vi "main.vi"() -> ()   [LabVIEW 2017]
uses:
  <vilib>/MakerHub/LINX/Public/Utilities/Open Serial.vi
  <vilib>/MakerHub/LINX/LMH-LINX.lvlib
panel:
  out "串口指示灯":bool
  out "成绩表":string[][](table)
  out "布尔":bool
  in  "硬件端口":refnum<visa-resource-name>="COM4"
  out "led1":bool
  out "黄绿色":bool
  out "绿色":bool
  out "蓝绿色":bool
  out "蓝色":bool
  out "蓝紫色":bool
  out "紫色":bool
  out "红紫色":bool
  out "品红":bool
  out "橙红色":bool
  out "橙色":bool
  out "黄橙色":bool
  out "黄色":bool
  out "led 12":bool
  out "led 11":bool
  out "led 10":bool
  out "led 9":bool
  out "led 8":bool
  out "led 7":bool
  out "led 6":bool
  out "led 5":bool
  out "led 4":bool
  out "led 3":bool
  out "led 2":bool
  out "Error Out":errorcluster
  out "B coff":dbl format="%.6f"
  out "G coff":dbl format="%.6f"
  out "R coff":dbl format="%.6f"
  in  "CAL":bool
  in  "学号":string="17101130123"
  in  "班级":string="视觉172"
  out "姓名":string
  in  "全体结束":bool
  in  "个人结束":bool
  in  "初始化":bool
  out "Blue":u8
  out "Green":u8
  out "Red":u8
  out "已答题数":u8(slide) scale=0.0..12.0
  out "stdcolour":u32[](array[colorbox])
  in  "boolcolour":bool[](array[boolean])
  out "error out":errorcluster caption="错误输出"
  in  "error in (no error)":errorcluster caption="错误输入（无错误）"
  out "已得分数":u8(slide) scale=0.0..100.0
  out "Color":u32(colorbox) caption="颜色"
  # "基于LabVIEW与颜色传感器的色环检测系统"
  # "黄色"
  # "黄橙色"
  # "橙色"
  # "橙红色"
  # "品红"
  # "红紫色"
  # "紫色"
  # "蓝紫色"
  # "蓝色"
  # "蓝绿色"
  # "绿色"
  # "黄绿色"
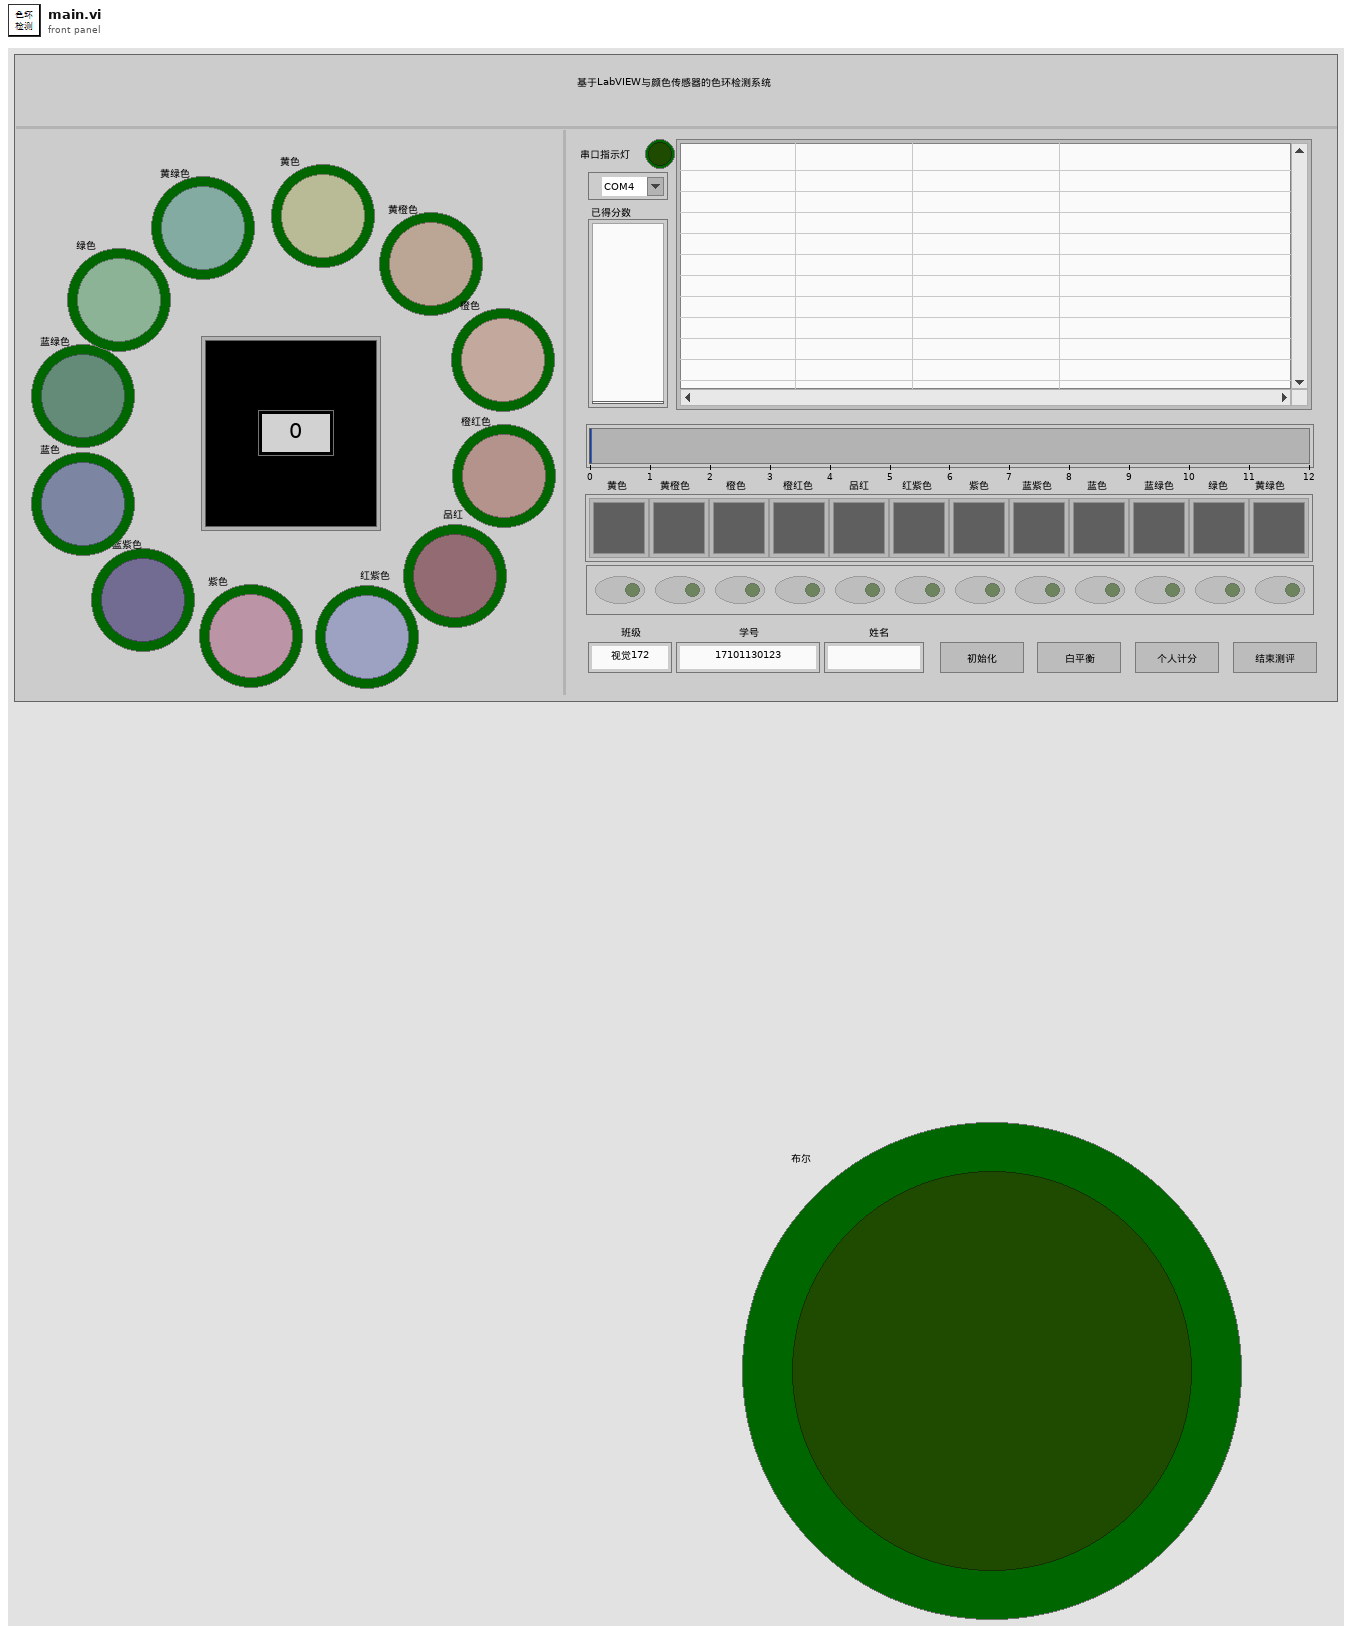
[diagram p1: front panel]
types:
  T1 = enum16{"open", "replace", "create", "open or create", "replace or create", "replace or create with confirmation"}
  T2 = typedef "LMH-LINX.lvlib/LINX Ref.ctl" = cluster{"IO":T3, "Interface":T4, "LINX Device Config":T5}
  T3 = typedef "LMH-LINX.lvlib/Platform.ctl" = enum16{"Remote", "Local"}
  T4 = typedef "LMH-LINX.lvlib/Interface.ctl" = enum16{"Serial", "TCP"}
  T5 = typedef "LMH-LINX.lvlib/Device.lvlib/LINX Device Config.ctl" = cluster{"Interface":T4, "COM Port":refnum<visa-resource-name>, "TCP Configuration":T6, "Device Family":u8, "Device ID":u8, "Device Name":string, "TCP Ref":refnum<k5>, "Channels":T7}
  T6 = typedef "LMH-LINX.lvlib/Device.lvlib/TCP Config.ctl" = cluster{"IP Address":string, "Port":u16}
  T7 = typedef "LMH-LINX.lvlib/Channels.ctl" = cluster{"DI":u8[], "DO":u8[], "AI":u8[], "AO":u8[], "PWM":u8[], "QE":u8[], "UART":u8[], "I2C 2":u8[], "SPI":u8[], "CAN":u8[], "Servo":u8[], "AI Ref (V)":dbl, "AI Resolution (Bits)":u8, "AO Ref (V)":dbl, "AO Resolution (Bits)":u8}
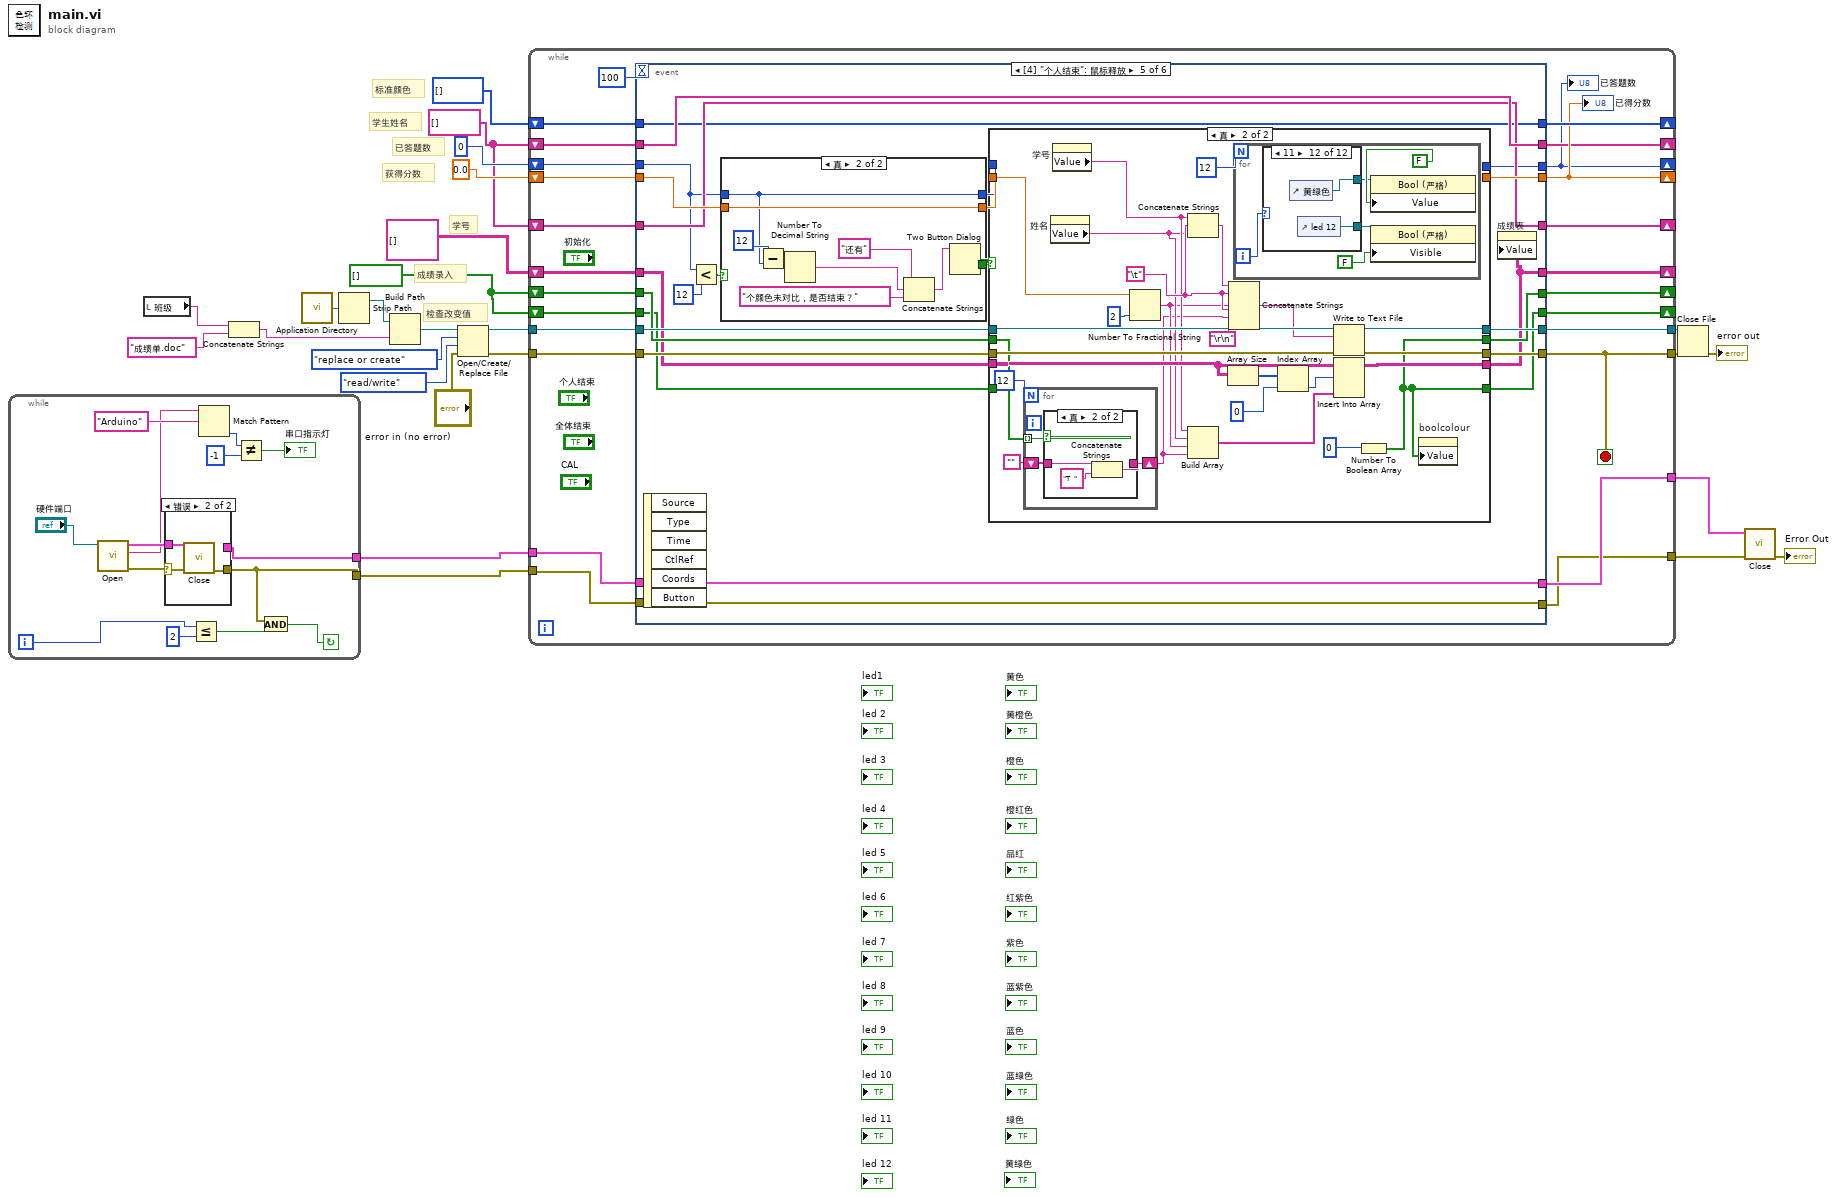
[diagram p0: block diagram]
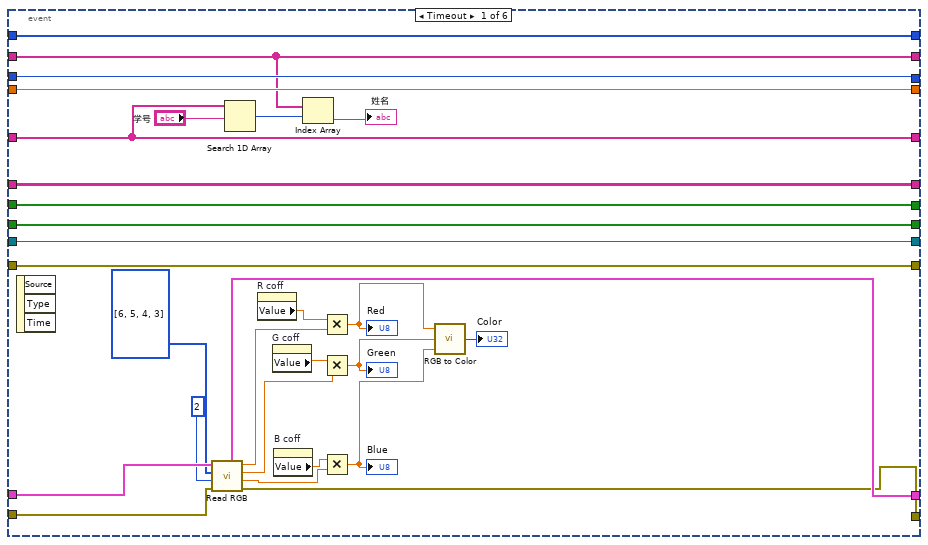
[diagram p3: hidden frame]
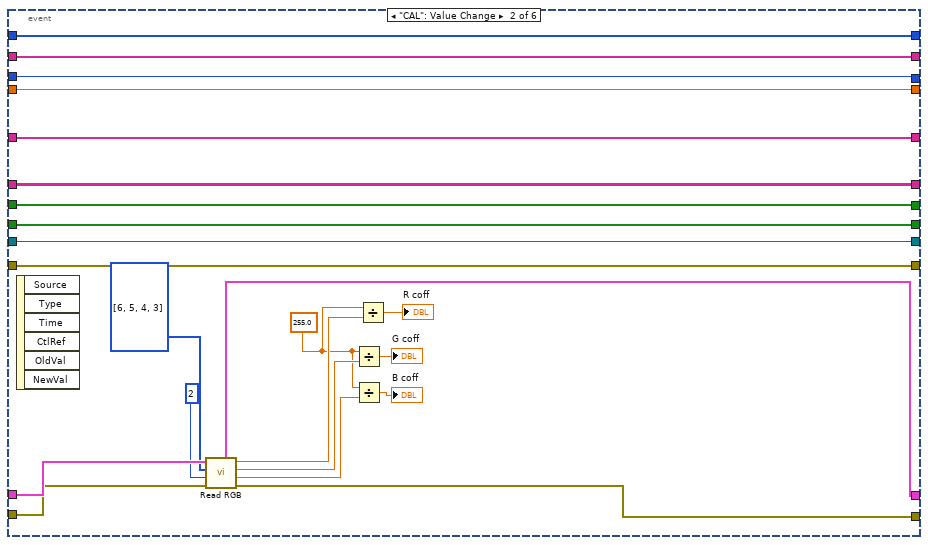
[diagram p4: hidden frame]
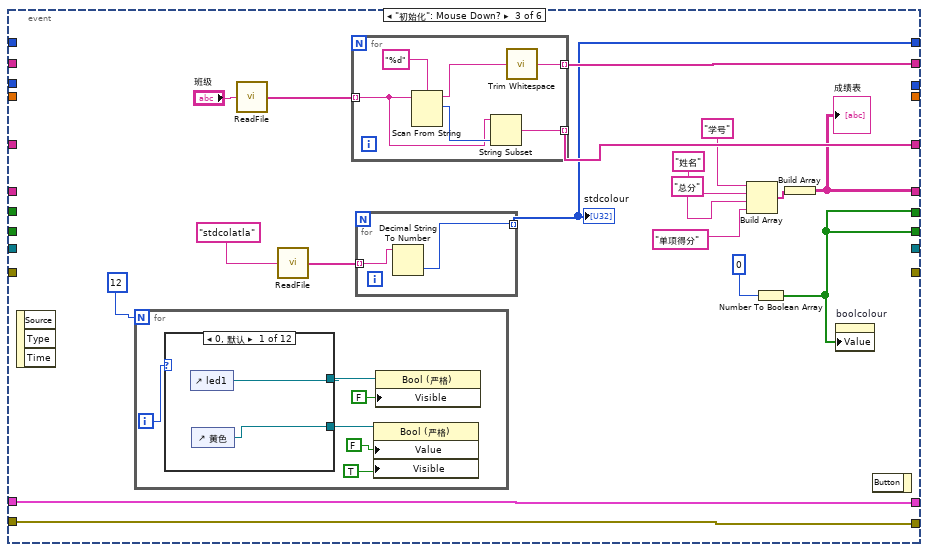
[diagram p5: hidden frame]
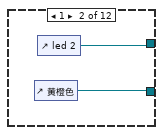
[diagram p6: hidden frame]
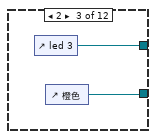
[diagram p7: hidden frame]
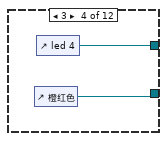
[diagram p8: hidden frame]
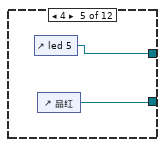
[diagram p9: hidden frame]
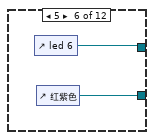
[diagram p10: hidden frame]
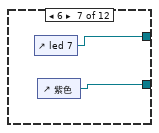
[diagram p11: hidden frame]
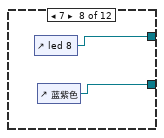
[diagram p12: hidden frame]
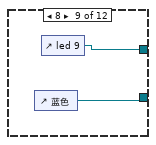
[diagram p13: hidden frame]
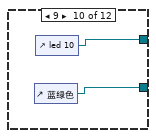
[diagram p14: hidden frame]
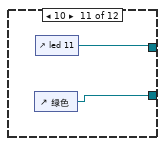
[diagram p15: hidden frame]
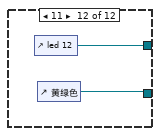
[diagram p16: hidden frame]
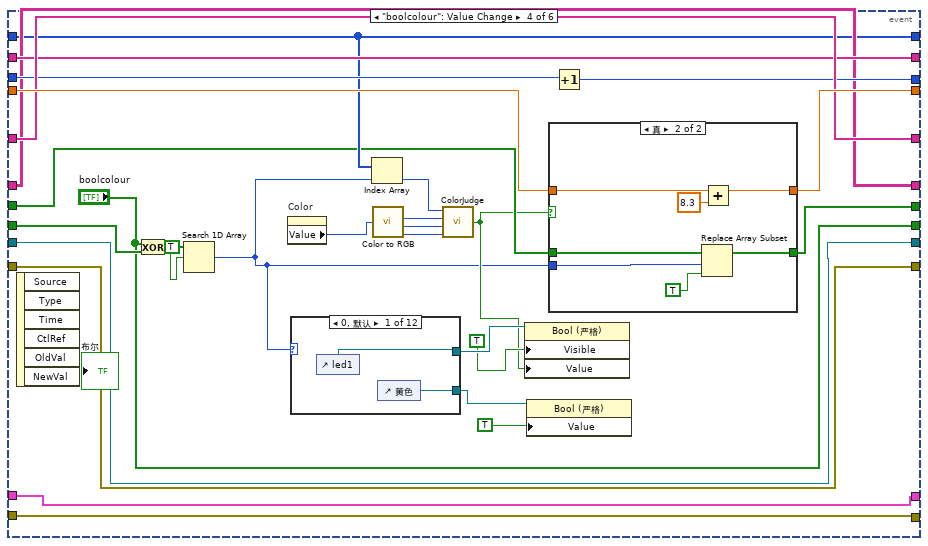
[diagram p17: hidden frame]
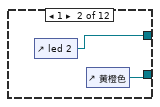
[diagram p18: hidden frame]
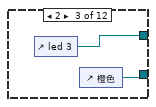
[diagram p19: hidden frame]
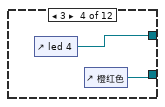
[diagram p20: hidden frame]
diagram:
  w10 = bool[] []
  w11 = string[] []
  # "检查改变值"
  # "成绩录入"
  # "已答题数"
  # "学号"
  # "获得分数"
  # "学生姓名"
  # "标准颜色"
  n1 = while {
    tunnel: [w36] -> w8
    tunnel: [w35] -> w5
    i -> [w34]
    stop <- w31 continue-if-true
    n2 = call-poly <vilib>:"Open.vi"("Serial Port"="硬件端口") -> ("Error Out"=w38:errorcluster, "Device Name"=w27:string, "LINX Resource"=w37:T2)  [unwired: 8 in]
    n3 = case shown="错误" w38 {
      selector: w38 -> [w40 w43]
      tunnel: w37 -> [w41 w42]
      tunnel: [w41 _] -> w36
      tunnel: [w40 w44] -> w35
      frame No Error {
      }
      frame Error {
        n4 = call <vilib>:"Close.vi"("Error In"=w43, "LINX Resource"=w42) -> ("Error Out"=w44:errorcluster)  [unwired: 9 in]
      }
    }
    n5 = Less Or Equal?(x=w34, y=2) -> (x <= y?=w32:bool)
    n6 = Match Pattern(string=w27, regular expression="Arduino" ("格式字符串")) -> (offset past match=w29:i32)  [unwired: 1 in, 3 out]
    n7 = Not Equal?(x=w29, y=-1) -> (x != y?=→"串口指示灯":bool)
    n8 = And(x=w35, y=w32) -> (x .and. y?=w31:bool)
  }
  n9 = local read "班级"() -> (w3:string)
  n10 = Concatenate Strings(w3, "成绩单.doc" ("名称或相对路径")) -> (w1:string)
  n11 = call <vilib>:"Application Directory.vi"() -> ("Application Directory"=w24:path)
  n12 = Strip Path(path=w24) -> (stripped path=w23:path)  [unwired: 1 out]
  n13 = Build Path(base path=w23, name or relative path=w1) -> (appended path=w22:path)
  n14 = Open/Create/Replace File(file path (use dialog)=w22, error in="error in (no error)", operation (0:open)=T1."replace or create" ("操作(0:open)"), access (0:read/write)=enum16{"read/write", "read-only", "write-only"}."read/write" ("权限(0:read/write)")) -> (refnum out=w19:refnum<file>, error out=w18:errorcluster)  [unwired: 2 in, 1 out]
  n15 = while {
    shift-right: [w69] -> _
    shift-left: i32[] [] -> [w68]
    tunnel: w19 -> [w51]
    tunnel: w18 -> [w67]
    tunnel: [w65] -> w16
    tunnel: [w66] -> w17
    shift-right: [w63] -> _
    shift-left: 0.0 -> [w64]
    shift-right: [w61] -> _
    shift-left: w11 -> [w60]
    shift-right: [w62] -> _
    shift-left: w11 -> [w59]
    shift-right: [w57] -> _
    shift-left: w10 -> [w58]
    shift-right: [w52] -> _
    shift-left: 0 -> [w56]
    shift-right: [w45] -> _
    shift-left: string[][] [] -> [w55]
    shift-right: [w53] -> _
    shift-left: w10 -> [w54]
    tunnel: w8 -> [w50]
    tunnel: [w49] -> w7
    tunnel: [w48] -> w6
    tunnel: w5 -> [w47]
    stop <- w66 stop-if-true
    n16 = event shown="[4] \"个人结束\": 鼠标释放" {
      selector: _ -> [_ _ _ _ _ _]
      dyn-events: _ -> [_ _ _ _ _ _]
      timeout: 100 -> [_ _ _ _ _ _]
      tunnel: [w98 w121 w133 w191 w243 _] -> w69
      tunnel: w68 -> [w98 w121 _ w191 w243 _]
      tunnel: w67 -> [w91 w112 _ w192 w262 _]
      tunnel: [w91 w112 _ w192 w261 errorcluster {"status"=TRUE, "code"=0, "source"=""} ("error in (no error) 2")] -> w66
      tunnel: [w92 w113 _ w193 w260 _] -> w65
      tunnel: w51 -> [w92 w113 _ w193 w259 _]
      tunnel: w64 -> [w96 w118 _ w203 w255 _]
      tunnel: [w96 w118 _ w202 w257 _] -> w63
      tunnel: [w71 w120 w137 w200 w253 _] -> w61
      tunnel: [w73 w117 w136 w201 w252 _] -> w62
      tunnel: w60 -> [w71 w120 _ w200 w253 _]
      tunnel: w59 -> [w73 w117 _ w201 w252 _]
      tunnel: w58 -> [w94 w115 _ w189 w251 _]
      tunnel: [w94 w115 w125 w188 w250 _] -> w57
      tunnel: w56 -> [w97 w119 _ w199 w249 _]
      tunnel: [w97 w119 _ w198 w248 _] -> w52
      tunnel: w55 -> [w95 w116 _ w197 w246 w349]
      tunnel: [w95 w116 w122 w197 w240 w349] -> w45
      tunnel: w54 -> [w93 w114 _ w196 w245 _]
      tunnel: [w93 w114 w125 "boolcolour" w244 _] -> w53
      tunnel: w50 -> [w83 w104 w124 w183 w242 w348]
      tunnel: [w80 w100 w124 w183 w242 w348] -> w49
      tunnel: [w79 w99 w123 w182 w241 w347] -> w48
      tunnel: w47 -> [w78 w103 w123 w182 w241 w347]
      event Timeout {
        n17 = event-data() -> ()  [unwired: 1 in, 3 out]
        n18 = call "Read RGB.vi"("错误输入（无错误）"=w78, "Pulse OUT"=u8 2, "S0S1S2S3"=u8[] [6, 5, 4, 3] ("DO Channels"), "LINX Resource输入"=w83) -> ("错误输出"=w79:errorcluster, "Blue"=w88:dbl, "Green"=w89:dbl, "Red"=w90:dbl, "LINX Resource输出"=w80:T2)  [unwired: 3 in]
        n19 = Search 1D Array(1D array=w73, element="学号") -> (index of element=w72:i32)  [unwired: 1 in]
        n20 = property on="R coff" class="DigNum (严格)"() -> ("Value"=w77:dbl)  [unwired: 2 in, 2 out]
        n21 = property on="G coff" class="DigNum (严格)"() -> ("Value"=w76:dbl)  [unwired: 2 in, 2 out]
        n22 = property on="B coff" class="DigNum (严格)"() -> ("Value"=w75:dbl)  [unwired: 2 in, 2 out]
        n23 = Index Array(array=w71, index=w72) -> (element=→"姓名":string)
        n24 = Multiply(x=w77, y=w90) -> (x*y=w86:dbl)
        "Red" <- w86
        n25 = Multiply(x=w76, y=w89) -> (x*y=w85:dbl)
        "Green" <- w85
        n26 = Multiply(x=w75, y=w88) -> (x*y=w84:dbl)
        "Blue" <- w84
        n27 = call <vilib>:"RGB to Color.vi"("B"=w84, "G"=w85, "R"=w86) -> ("Color"=→"Color":u32)
      }
      event "CAL": Value Change {
        w108 = 255.0 ("x")
        n28 = event-data() -> ()  [unwired: 1 in, 6 out]
        n29 = call "Read RGB.vi"("错误输入（无错误）"=w103, "Pulse OUT"=u8 2, "S0S1S2S3"=u8[] [6, 5, 4, 3] ("DO Channels"), "LINX Resource输入"=w104) -> ("错误输出"=w99:errorcluster, "Blue"=w109:dbl, "Green"=w110:dbl, "Red"=w111:dbl, "LINX Resource输出"=w100:T2)  [unwired: 3 in]
        n30 = Divide(x=w108, y=w110) -> (x/y=→"G coff":dbl)
        n31 = Divide(x=w108, y=w109) -> (x/y=→"B coff":dbl)
        n32 = Divide(x=w108, y=w111) -> (x/y=→"R coff":dbl)
      }
      event "初始化": Mouse Down? {
        n33 = event-data() -> ()  [unwired: 1 in, 3 out]
        n34 = for {
          N: 12 -> [_]
          i -> [w145]
          n35 = case shown="0, 默认" w145 {
            tunnel: [w147 w149 w151 w153 w155 w157 w159 w161 w163 w165 w167 w169] -> w144
            tunnel: [w146 w148 w150 w152 w154 w156 w158 w160 w162 w164 w166 w168] -> w142
            frame 0, Default {
              n36 = control-ref of="led1"() -> (w147:refnum<vi>)
              n37 = control-ref of="黄色"() -> (w146:refnum<vi>)
            }
            frame 1 {
              n38 = control-ref of="黄橙色"() -> (w148:refnum<vi>)
              n39 = control-ref of="led 2"() -> (w149:refnum<vi>)
            }
            frame 2 {
              n40 = control-ref of="led 3"() -> (w151:refnum<vi>)
              n41 = control-ref of="橙色"() -> (w150:refnum<vi>)
            }
            frame 3 {
              n42 = control-ref of="橙红色"() -> (w152:refnum<vi>)
              n43 = control-ref of="led 4"() -> (w153:refnum<vi>)
            }
            frame 4 {
              n44 = control-ref of="led 5"() -> (w155:refnum<vi>)
              n45 = control-ref of="品红"() -> (w154:refnum<vi>)
            }
            frame 5 {
              n46 = control-ref of="led 6"() -> (w157:refnum<vi>)
              n47 = control-ref of="红紫色"() -> (w156:refnum<vi>)
            }
            frame 6 {
              n48 = control-ref of="led 7"() -> (w159:refnum<vi>)
              n49 = control-ref of="紫色"() -> (w158:refnum<vi>)
            }
            frame 7 {
              n50 = control-ref of="led 8"() -> (w161:refnum<vi>)
              n51 = control-ref of="蓝紫色"() -> (w160:refnum<vi>)
            }
            frame 8 {
              n52 = control-ref of="蓝色"() -> (w162:refnum<vi>)
              n53 = control-ref of="led 9"() -> (w163:refnum<vi>)
            }
            frame 9 {
              n54 = control-ref of="蓝绿色"() -> (w164:refnum<vi>)
              n55 = control-ref of="led 10"() -> (w165:refnum<vi>)
            }
            frame 10 {
              n56 = control-ref of="绿色"() -> (w166:refnum<vi>)
              n57 = control-ref of="led 11"() -> (w167:refnum<vi>)
            }
            frame 11 {
              n58 = control-ref of="led 12"() -> (w169:refnum<vi>)
              n59 = control-ref of="黄绿色"() -> (w168:refnum<vi>)
            }
          }
          n60 = property class="Bool (严格)"(reference=w142, "Value"=FALSE, "Visible"=TRUE) -> ()  [unwired: 1 in, 2 out]
          n61 = property class="Bool (严格)"(reference=w144, "Visible"=FALSE ("可见")) -> ()  [unwired: 1 in, 2 out]
        }
        n62 = call "ReadFile.vi"("文件名"="班级") -> ("文件内容"=w138:string[])
        n63 = call "ReadFile.vi"("文件名"="stdcolatla") -> ("文件内容"=w135:string[])
        n64 = for {
          tunnel: w138 -> [w172] mode=indexing
          tunnel: [w176] -> w137 mode=indexing
          tunnel: [w174] -> w136 mode=indexing
          n65 = Scan From String(format string="%d", input string=w172) -> (remaining string=w175:string, offset past scan=w173:u32)  [unwired: 4 in, 1 out]
          n66 = String Subset(string=w172, length (rest)=w173) -> (substring=w174:string)  [unwired: 1 in]
          n67 = call <vilib>:"Trim Whitespace.vi"("string"=w175) -> ("trimmed string"=w176:string)  [unwired: 1 in]
        }
        n68 = for {
          tunnel: w135 -> [w171] mode=indexing
          tunnel: [w170] -> w133 mode=indexing
          n69 = Decimal String To Number(string=w171) -> (number=w170:i32)  [unwired: 2 in, 1 out]
        }
        "stdcolour" <- w133
        n70 = Build Array("学号", "姓名", "总分", "单项得分") -> (w128:string[])
        n71 = Number To Boolean Array(number=0) -> (Boolean array=w125:bool[])
        n72 = Build Array(w128) -> (w122:string[][])
        "成绩表" <- w122
        n73 = property on="boolcolour" class="Arr (严格)"("Value"=w125) -> ()  [unwired: 2 in, 2 out]
        n74 = event-data() -> ()  [unwired: 2 in, 1 out]
      }
      event "boolcolour": Value Change {
        n75 = event-data() -> ()  [unwired: 1 in, 6 out]
        n76 = Exclusive Or(1:w196, 2:"boolcolour") -> (0:w195:bool[])
        n77 = Search 1D Array(1D array=w195, element=TRUE) -> (index of element=w178:i32)  [unwired: 1 in]
        n78 = property on="Color" class="ColBox"() -> ("Value"=w184:u32)  [unwired: 2 in, 2 out]
        n79 = case shown="0, 默认" w178 {
          tunnel: [w208 w210 w212 w214 w216 w218 w220 w222 w224 w226 w228 w230] -> w186
          tunnel: [w207 w209 w211 w213 w215 w217 w219 w221 w223 w225 w227 w229] -> w180
          frame 0, Default {
            n80 = control-ref of="led1"() -> (w208:refnum<vi>)
            n81 = control-ref of="黄色"() -> (w207:refnum<vi>)
          }
          frame 1 {
            n82 = control-ref of="led 2"() -> (w210:refnum<vi>)
            n83 = control-ref of="黄橙色"() -> (w209:refnum<vi>)
          }
          frame 2 {
            n84 = control-ref of="led 3"() -> (w212:refnum<vi>)
            n85 = control-ref of="橙色"() -> (w211:refnum<vi>)
          }
          frame 3 {
            n86 = control-ref of="led 4"() -> (w214:refnum<vi>)
            n87 = control-ref of="橙红色"() -> (w213:refnum<vi>)
          }
          frame 4 {
            n88 = control-ref of="led 5"() -> (w216:refnum<vi>)
            n89 = control-ref of="品红"() -> (w215:refnum<vi>)
          }
          frame 5 {
            n90 = control-ref of="led 6"() -> (w218:refnum<vi>)
            n91 = control-ref of="红紫色"() -> (w217:refnum<vi>)
          }
          frame 6 {
            n92 = control-ref of="led 7"() -> (w220:refnum<vi>)
            n93 = control-ref of="紫色"() -> (w219:refnum<vi>)
          }
          frame 7 {
            n94 = control-ref of="led 8"() -> (w222:refnum<vi>)
            n95 = control-ref of="蓝紫色"() -> (w221:refnum<vi>)
          }
          frame 8 {
            n96 = control-ref of="led 9"() -> (w224:refnum<vi>)
            n97 = control-ref of="蓝色"() -> (w223:refnum<vi>)
          }
          frame 9 {
            n98 = control-ref of="led 10"() -> (w226:refnum<vi>)
            n99 = control-ref of="蓝绿色"() -> (w225:refnum<vi>)
          }
          frame 10 {
            n100 = control-ref of="led 11"() -> (w228:refnum<vi>)
            n101 = control-ref of="绿色"() -> (w227:refnum<vi>)
          }
          frame 11 {
            n102 = control-ref of="led 12"() -> (w230:refnum<vi>)
            n103 = control-ref of="黄绿色"() -> (w229:refnum<vi>)
          }
        }
        n104 = Index Array(array=w191, index=w178) -> (element=w190:i32)
        n105 = call <vilib>:"Color to RGB.vi"("Color"=w184) -> ("R"=w206:u8, "G"=w205:u8, "B"=w204:u8)  [unwired: 1 out]
        n106 = call "ColorJudge.vi"("B"=w204, "G"=w205, "R"=w206, "C"=w190) -> ("out"=w181:bool)
        n107 = property class="Bool (严格)"(reference=w186, "Visible"=TRUE, "Value"=w181) -> ()  [unwired: 1 in, 2 out]
        n108 = property class="Bool (严格)"(reference=w180, "Value"=TRUE) -> ()  [unwired: 1 in, 2 out]
        n109 = case shown="真" w181 {
          tunnel: w203 -> [w232 w239]
          tunnel: [w232 w237] -> w202
          tunnel: w189 -> [w231 w236]
          tunnel: [w231 w233] -> w188
          tunnel: w178 -> [_ w235]
          frame False {
          }
          frame True {
            n110 = Replace Array Subset(array=w236, new element=TRUE, index=w235) -> (w233:bool[])
            n111 = Add(x=w239, y=8.3) -> (x+y=w237:dbl)
          }
        }
        n112 = Increment(x=w199) -> (x+1=w198:i32)
      }
      event "个人结束": Mouse Up {
        n113 = event-data() -> ()  [unwired: 1 in, 6 out]
        n114 = Less?(x=w249, y=12) -> (x < y?=w258:bool)
        n115 = case shown="真" w258 {
          tunnel: [w265 w269] -> w256
          tunnel: w255 -> [w265 w269]
          tunnel: [TRUE w268] -> w254
          tunnel: w249 -> [w264 w267]
          tunnel: [w264 w267] -> w247
          frame False {
          }
          frame True {
            n116 = Subtract(x=12, y=w267) -> (x-y=w274:i32)
            n117 = Number To Decimal String(number=w274) -> (decimal integer string=w271:string)  [unwired: 1 in]
            n118 = Concatenate Strings("还有", w271, "个颜色未对比，是否结束？") -> (w270:string)
            n119 = Two Button Dialog(message=w270) -> (T button?=w268:bool)  [unwired: 2 in]
          }
        }
        n120 = case shown="真" w254 {
          tunnel: w262 -> [w281 w304]
          tunnel: [w281 w306] -> w261
          tunnel: [w282 w307] -> w260
          tunnel: w259 -> [w282 w305]
          tunnel: [w280 _] -> w257
          tunnel: w256 -> [w280 w303]
          tunnel: w251 -> [w279 w298]
          tunnel: [w279 w285] -> w250
          tunnel: [w278 _] -> w248
          tunnel: w247 -> [w278 _]
          tunnel: w246 -> [w277 w300]
          tunnel: [w277 w299] -> w240
          tunnel: w245 -> [w276 _]
          tunnel: [w276 w285] -> w244
          frame False {
          }
          frame True {
            w296 = "\t"
            n121 = for {
              N: 12 -> [_]
              tunnel: w298 -> [w340] mode=indexing
              shift-right: [w338] -> w289
              shift-left: "" -> [w339]
              n122 = case shown="真" w340 {
                tunnel: w339 -> [w343 w346]
                tunnel: [w342 w344] -> w338
                frame False {
                  n123 = Concatenate Strings(w343, "F  ") -> (w342:string)
                }
                frame True {
                  n124 = Concatenate Strings(w346, "T  ") -> (w344:string)
                }
              }
            }
            n125 = property on="姓名" class="Str"() -> ("Value"=w291:string)  [unwired: 2 in, 2 out]
            n126 = property on="学号" class="Str"() -> ("Value"=w292:string)  [unwired: 2 in, 2 out]
            n127 = Number To Fractional String(number=w303, precision (6)=i16 2 ("精度(6)")) -> (F-format string=w290:string)  [unwired: 2 in]
            n128 = Concatenate Strings(w292, w296, w291) -> (w302:string)
            n129 = Build Array(w292, w291, w290, w289) -> (w288:string[])
            n130 = Array Size(array=w300) -> (size(s)=w294:i32[])
            n131 = Concatenate Strings(w302, w296, w290, w296, w289, "\r\n") -> (w301:string)
            n132 = for {
              N: 12 -> [_]
              i -> [w313]
              n133 = case shown="11" w313 {
                tunnel: [w315 w317 w319 w321 w323 w325 w327 w329 w331 w333 w335 w337] -> w312
                tunnel: [w314 w316 w318 w320 w322 w324 w326 w328 w330 w332 w334 w336] -> w309
                frame 0, Default {
                  n134 = control-ref of="led1"() -> (w315:refnum<vi>)
                  n135 = control-ref of="黄色"() -> (w314:refnum<vi>)
                }
                frame 1 {
                  n136 = control-ref of="黄橙色"() -> (w316:refnum<vi>)
                  n137 = control-ref of="led 2"() -> (w317:refnum<vi>)
                }
                frame 2 {
                  n138 = control-ref of="橙色"() -> (w318:refnum<vi>)
                  n139 = control-ref of="led 3"() -> (w319:refnum<vi>)
                }
                frame 3 {
                  n140 = control-ref of="橙红色"() -> (w320:refnum<vi>)
                  n141 = control-ref of="led 4"() -> (w321:refnum<vi>)
                }
                frame 4 {
                  n142 = control-ref of="品红"() -> (w322:refnum<vi>)
                  n143 = control-ref of="led 5"() -> (w323:refnum<vi>)
                }
                frame 5 {
                  n144 = control-ref of="红紫色"() -> (w324:refnum<vi>)
                  n145 = control-ref of="led 6"() -> (w325:refnum<vi>)
                }
                frame 6 {
                  n146 = control-ref of="紫色"() -> (w326:refnum<vi>)
                  n147 = control-ref of="led 7"() -> (w327:refnum<vi>)
                }
                frame 7 {
                  n148 = control-ref of="蓝紫色"() -> (w328:refnum<vi>)
                  n149 = control-ref of="led 8"() -> (w329:refnum<vi>)
                }
                frame 8 {
                  n150 = control-ref of="蓝色"() -> (w330:refnum<vi>)
                  n151 = control-ref of="led 9"() -> (w331:refnum<vi>)
                }
                frame 9 {
                  n152 = control-ref of="蓝绿色"() -> (w332:refnum<vi>)
                  n153 = control-ref of="led 10"() -> (w333:refnum<vi>)
                }
                frame 10 {
                  n154 = control-ref of="绿色"() -> (w334:refnum<vi>)
                  n155 = control-ref of="led 11"() -> (w335:refnum<vi>)
                }
                frame 11 {
                  n156 = control-ref of="黄绿色"() -> (w336:refnum<vi>)
                  n157 = control-ref of="led 12"() -> (w337:refnum<vi>)
                }
              }
              n158 = property class="Bool (严格)"(reference=w309, "Value"=FALSE) -> ()  [unwired: 1 in, 2 out]
              n159 = property class="Bool (严格)"(reference=w312, "Visible"=FALSE) -> ()  [unwired: 1 in, 2 out]
            }
            n160 = Index Array(array=w294, index=0) -> (element=w293:i32)
            n161 = Write to Text File(file (use dialog)=w305, text=w301, error in=w304) -> (refnum out=w307:refnum<file>, error out=w306:errorcluster)  [unwired: 1 in, 1 out]
            n162 = Insert Into Array(array=w300, index (row)=w293, new element=w288) -> (w299:string[][])  [unwired: 1 in]
            n163 = Number To Boolean Array(number=0) -> (Boolean array=w285:bool[])
            n164 = property on="boolcolour" class="Arr (严格)"("Value"=w285) -> ()  [unwired: 2 in, 2 out]
          }
        }
        n165 = property on="成绩表" class="Tbl (严格)"("Value"=w240) -> ()  [unwired: 2 in, 2 out]
      }
      event "全体结束": Mouse Down? {
        n166 = event-data() -> ()  [unwired: 1 in, 3 out]
        n167 = event-data() -> ()  [unwired: 2 in, 1 out]
      }
    }
    "已得分数" <- w63
    "已答题数" <- w52
  }
  n168 = Close File(refnum=w16, error in=w17) -> (error out=→"error out":errorcluster)  [unwired: 1 out]
  n169 = call <vilib>:"Close.vi"("Error In"=w6, "LINX Resource"=w7) -> ("Error Out"=→"Error Out":errorcluster)  [unwired: 9 in]
